vi "InitCan.vi"(8 "VCI_INIT_CONFIG":T1={"AccCode"=52428, "AccMask"=16777215, "Reserved"=222222, "Filter"=0, "Timing0"=1, "Timing1"=28, "Mode"=0} {"AccCode" format="%x"; "AccMask" format="%x"; "Reserved" format="%x"; "Timing1" format="%x"}, 9 "CanIndex_IN":u32, 10 "DevIndex_IN":u32, 11 "DevType_IN":u32) -> (1 "CanIndex_OUT":u32, 2 "DevIndex_OUT":u32, 3 "DevType_OUT":u32, 5 "InitCAN_Success?":u32)   [LabVIEW 2016]
uses:
  ECanVci.dll
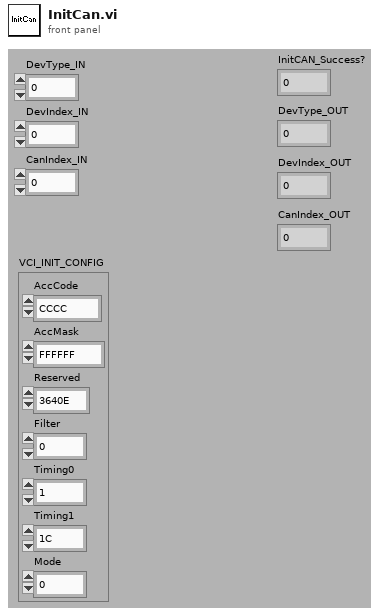
[diagram p1: front panel]
types:
  T1 = cluster{"AccCode":u32, "AccMask":u32, "Reserved":u32, "Filter":u8, "Timing0":u8, "Timing1":u8, "Mode":u8}
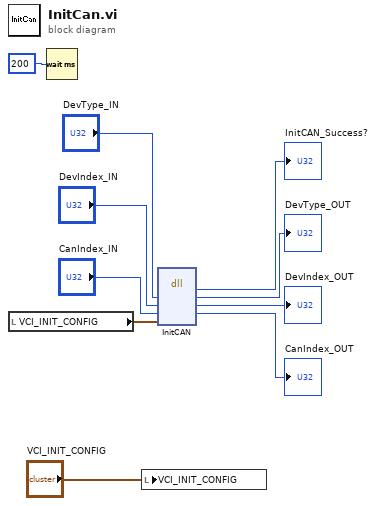
[diagram p0: block diagram]
diagram:
  n1 = local read "VCI_INIT_CONFIG"() -> (w1:T1)
  n2 = Wait (ms)(milliseconds to wait=u32 200 ("等待时间（毫秒）")) -> ()  [unwired: 1 out]
  n3 = local write "VCI_INIT_CONFIG"("VCI_INIT_CONFIG") -> ()
  n4 = dll-call lib="C:/Users/Azmat/Desktop/Labview/ECanVci.dll" fn="InitCAN"("DevType"="DevType_IN", "DevIndex"="DevIndex_IN", "CanIndex"="CanIndex_IN", "pInit_Config"=w1) -> ("InitCan_Success"=→"InitCAN_Success?":i32, "DevType"=→"DevType_OUT":u32, "DevIndex"=→"DevIndex_OUT":u32, "CanIndex"=→"CanIndex_OUT":u32)  [unwired: 4 in, 2 out]
